vi "fg_Pockels modulation data.vi"(9 "Pockels modulation data in":dbl[](array[numeric]), 11 "Function":T1) -> (1 "Pockels modulation data out":dbl[](array[numeric]))   [LabVIEW 2013]
uses:
  Typedefs/Functional Global Default States.ctl
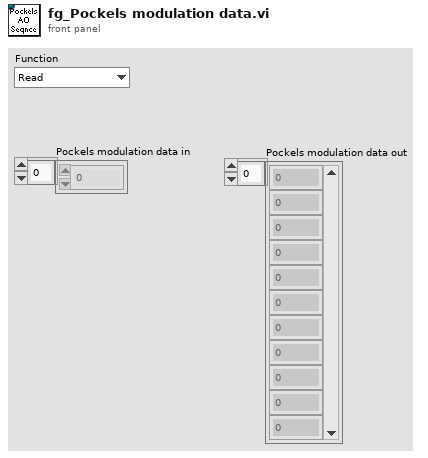
[diagram p1: front panel]
types:
  T1 = typedef "Functional Global Default States.ctl" = enum16{"Read", "Write", "Clear"}
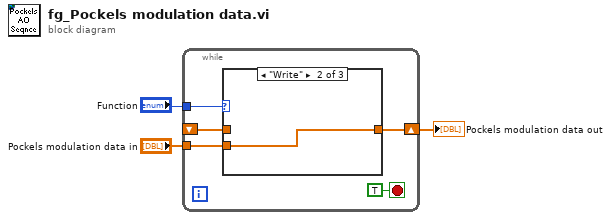
[diagram p0: block diagram]
diagram:
  n1 = while {
    shift-right: [w6] -> w2
    shift-left: _ -> [w8]
    tunnel: "Pockels modulation data in" -> [w7]
    tunnel: "Function" -> [w4]
    stop <- TRUE stop-if-true
    n2 = case shown="\"Write\"" w4 {
      tunnel: w8 -> [w9 _ _]
      tunnel: w7 -> [_ w10 _]
      tunnel: [w9 w10 _] -> w6
      frame "Read", Default {
      }
      frame "Write" {
      }
      frame "Clear" {
      }
    }
  }
  "Pockels modulation data out" <- w2
